vi "Demo - Read 1 Analog Input Continuously.vi"() -> ()   [LabVIEW 2021]
uses:
  TypeDefs/Enum - Machine State.ctl
  TypeDefs/TypeDef - Cluster of DAQiFi Device Properties.ctl
  TypeDefs/Enum - Connection Type.ctl
  <vilib>/ErrorRing/Error Ring.xnode
panel:
  out "Program Status":string
  in  "Stop":bool
  out "Waveform Chart":dbl(graph)
  in  "DAQ IP Address or COM Port":string="192.168.1.1"
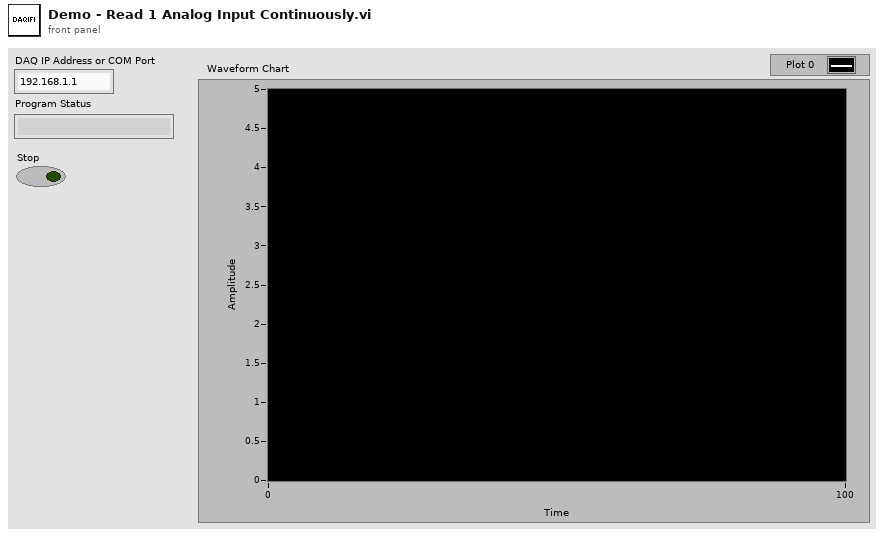
[diagram p1: front panel]
types:
  T1 = typedef "TypeDef - Cluster of DAQiFi Device Properties.ctl" = cluster{"IP Address":string, "MAC Address":string, "Serial Number":string, "Connection Type":T2, "Connected":bool, "TCP Network Connection":refnum<k5>, "USB Serial Connection":refnum<visa-resource-name>}
  T2 = typedef "Enum - Connection Type.ctl" = enum16{"USB", "TCP"}
  T3 = typedef "Enum - Machine State.ctl" = enum16{"Shutdown", "Save Data", "Start Streaming", "Initialize", "Read Streamed Data"}
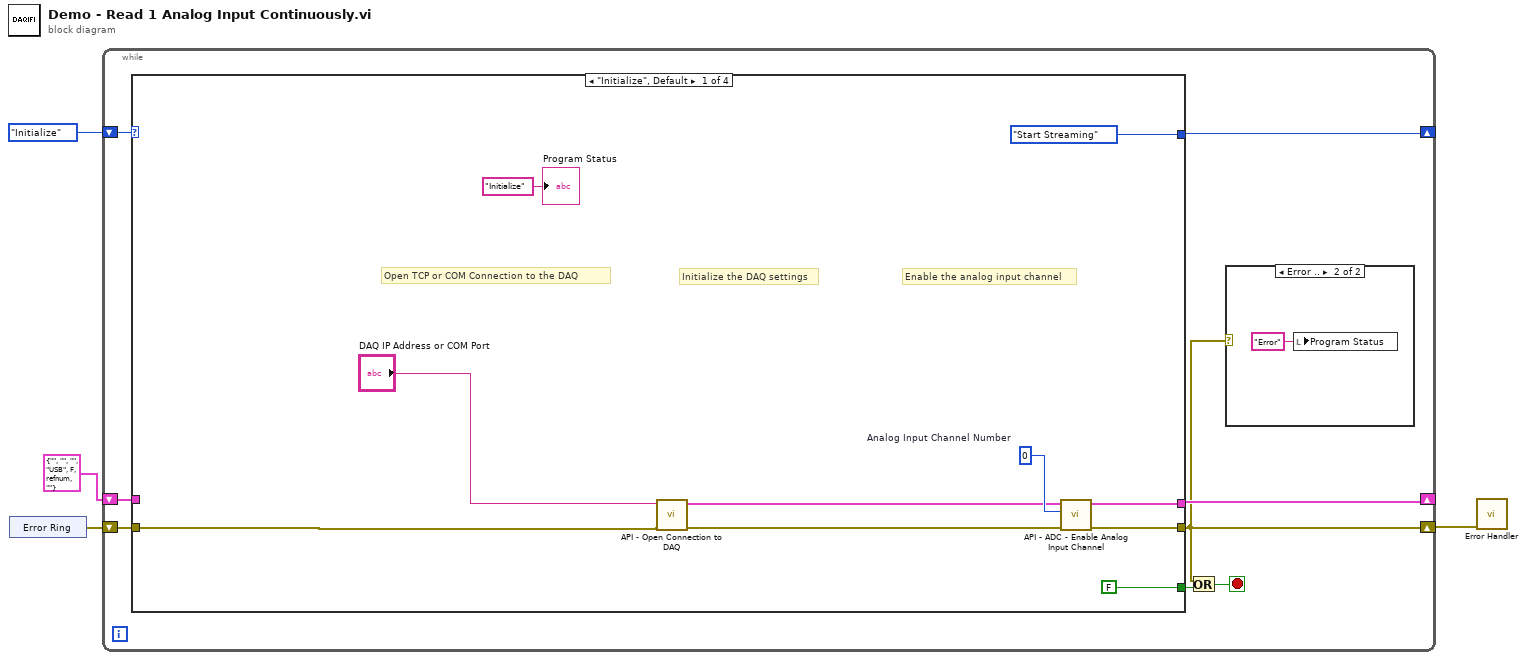
[diagram p0: block diagram]
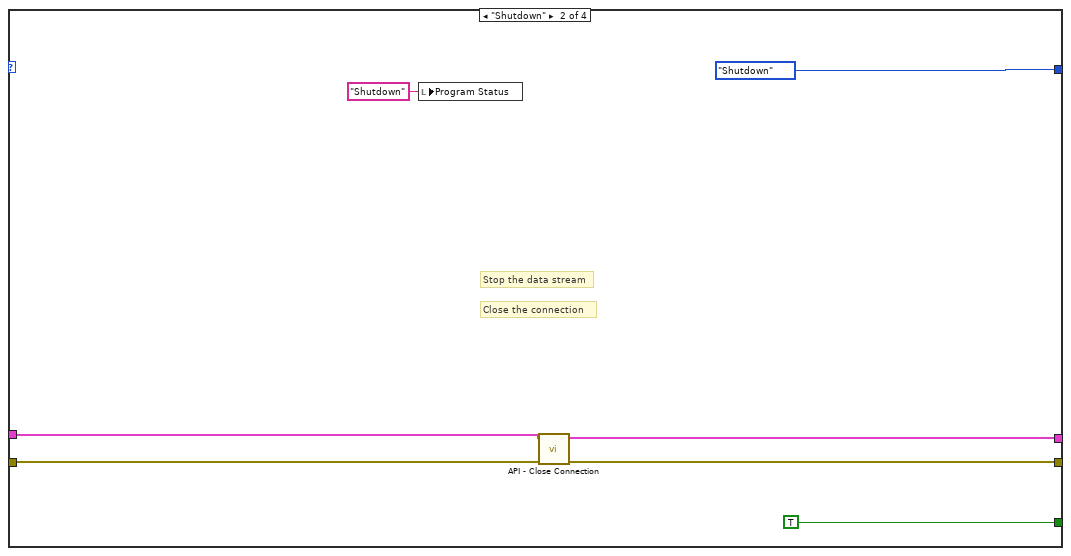
[diagram p3: hidden frame]
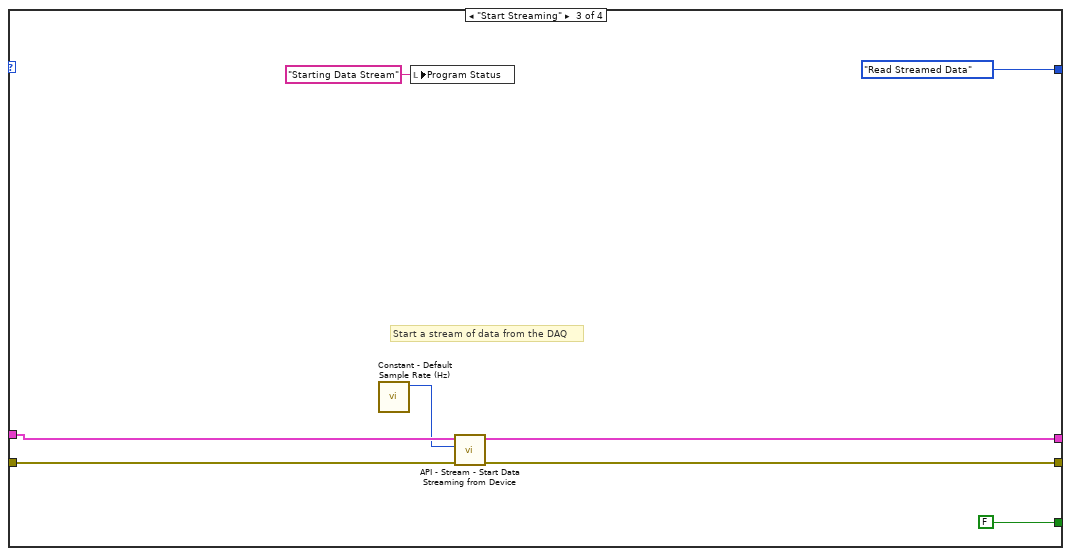
[diagram p4: hidden frame]
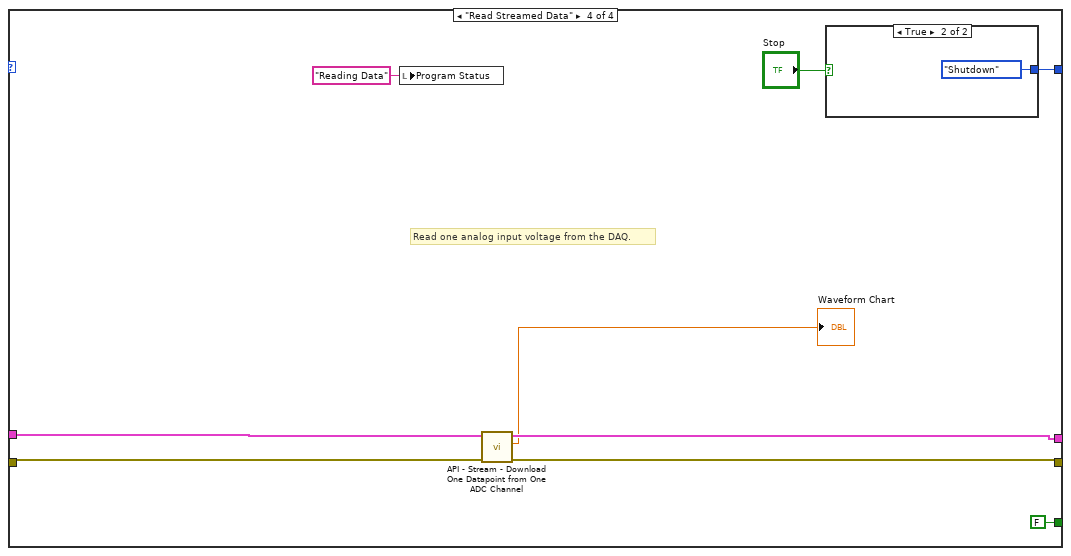
[diagram p5: hidden frame]
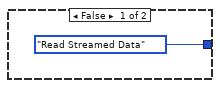
[diagram p6: hidden frame]
diagram:
  n1 = xnode "Error Ring"() -> ("error out"=w3:errorcluster)
  n2 = while {
    shift-right: [w5] -> w2
    shift-left: w3 -> [w11]
    shift-right: [w10] -> _
    shift-left: T1 {"IP Address"="", "MAC Address"="", "Serial Number"="", "Connection Type"=enum."USB", "Connected"=FALSE, "TCP Network Connection"=refnum, "USB Serial Connection"=""} ("DAQiFi Device Properties") -> [w8]
    shift-right: [w9] -> _
    shift-left: Enum_-_Machine_State."Initialize" -> [w12]
    stop <- w6 stop-if-true
    n3 = case shown="\"Initialize\", Default" w12 {
      tunnel: w11 -> [w15 w26 w32 w42]
      tunnel: [w20 w25 w33 w41] -> w5
      tunnel: [w21 w24 w34 w40] -> w10
      tunnel: [Enum_-_Machine_State."Start Streaming" Enum_-_Machine_State."Shutdown" Enum_-_Machine_State."Read Streamed Data" w47] -> w9
      tunnel: [FALSE TRUE FALSE FALSE] -> w7
      tunnel: w8 -> [_ w27 w35 w43]
      frame "Initialize", Default {
        w18 = 0  # Analog Input Channel Number
        # "Enable the analog input channel"
        # "Open TCP or COM Connection to the DAQ"
        # "Initialize the DAQ settings"
        n4 = call "API - Open Connection to DAQ.vi"("error in"=w15, "DAQ Address (IP or COM)"="DAQ IP Address or COM Port") -> ("error out"=w14:errorcluster, "DAQiFi Device Properties"=w16:T1)  [unwired: 8 in]
        n5 = call "API - ADC - Enable Analog Input Channel.vi"("error in (no error)"=w14, "Analog Input Channel Number"=w18, "DAQiFi Device Properties In"=w16) -> ("error out"=w20:errorcluster, "DAQiFi Device Properties Out"=w21:T1)  [unwired: 7 in]
        "Program Status" <- "Initialize" ("Program Status")
      }
      frame "Shutdown" {
        # "Close the connection"
        # "Stop the data stream"
        n6 = local write "Program Status"("Shutdown" ("Program Status")) -> ()
        n7 = call "API - Close Connection.vi"("error in"=w26, "DAQiFi Device Properties In"=w27) -> ("error out"=w25:errorcluster, "DAQiFi Device Properties Out"=w24:T1)  [unwired: 8 in]
      }
      frame "Start Streaming" {
        # "Start a stream of data from the DAQ"
        n8 = call "Constant - Default Sample Rate (Hz).vi"() -> ("Streaming Rate (Hz)"=w31:i32)  [unwired: 11 in]
        n9 = local write "Program Status"("Starting Data Stream" ("Program Status")) -> ()
        n10 = call "API - Stream - Start Data Streaming from Device.vi"("error in"=w32, "Streaming Rate (Hz)"=w31, "DAQiFi Device Properties In"=w35) -> ("error out"=w33:errorcluster, "DAQiFi Device Properties Out"=w34:T1)  [unwired: 7 in]
      }
      frame "Read Streamed Data" {
        # "Read one analog input voltage from the DAQ."
        n11 = local write "Program Status"("Reading Data" ("Program Status")) -> ()
        n12 = call "API - Stream - Download One Datapoint from One ADC Channel.vi"("error in"=w42, "DAQiFi Device Properties In"=w43) -> ("error out"=w41:errorcluster, "Analog Voltage (V)"=→"Waveform Chart":dbl, "DAQiFi Device Properties Out"=w40:T1)  [unwired: 7 in]
        n13 = case shown="True" "Stop" {
          tunnel: [Enum_-_Machine_State."Read Streamed Data" Enum_-_Machine_State."Shutdown"] -> w47
          frame False {
          }
          frame True {
          }
        }
      }
    }
    n14 = Or(x=w5, y=w7) -> (x .or. y?=w6:bool)
    n15 = case shown="Error .." w5 {
      frame No Error {
      }
      frame Error {
        n16 = local write "Program Status"("Error" ("Program Status")) -> ()
      }
    }
  }
  n17 = call "Error Handler.vi"("error in"=w2) -> ()  [unwired: 10 in, 1 out]
